vi "Sweep control.vi"(0 "Scan control":cluster{"Priority":u16, "Scan name":u16}[](array[cluster])=[{"Priority"=0, "Scan name"=1}, {"Priority"=1, "Scan name"=0}, {"Priority"=3, "Scan name"=0}, {"Priority"=2, "Scan name"=0}] {"Scan name" items=["OFF", "Vsg1", "Vsg2", "Vsgw", "Vbg", "Field", "Temp", "MW_freq", "MW_amplitude"]; "Priority" items=["Priority 0", "Priority 1", "Priority 2", "Priority 3", "Priority 4", "Priority 5"]}, 1 "Scan parameters":T2(array[cluster])=[{"DAQ Channel"=3, "Label"="\nappliedVsg=", "Scaled low"=-0.1, "Scaled high"=0.6, "Start"=-0.8, "End"=0.1, "Step"=0.001, "Scale?"=FALSE, "Output"=0}, {"DAQ Channel"=3, "Label"="\nappliedVsg2=", "Scaled low"=-0.175, "Scaled high"=0.775, "Start"=0.0, "End"=0.0, "Step"=0.01, "Scale?"=FALSE, "Output"=2}, {"DAQ Channel"=3, "Label"="\nappliedVbg=", "Scaled low"=-0.11, "Scaled high"=0.31, "Start"=-1.55, "End"=3.0, "Step"=0.015, "Scale?"=FALSE, "Output"=2}, {"DAQ Channel"=3, "Label"="\nappliedField=", "Scaled low"=-0.060000000000000005, "Scaled high"=0.14, "Start"=0.0, "End"=10000.0, "Step"=5000.0, "Scale?"=FALSE, "Output"=2}] {"Step" format="%#_6p"; "End" format="%#_6p"; "Start" format="%#_6p"; "Scaled high" format="%#_6p"; "Scaled low" format="%#_6p"}, 3 "Comments":string="SA02703G.20140721\n\nVbg=0.7V\n\nsweep Vsg2(control): -80mV to 100mV 1mV steps\n\nLockin0:18\n1: 19\n2: 21\n3: 22\n4: 23\n5: 24\n\ndrive differentially 18,24, 1mV 401mHz", 4 "Experiment folder name":string="1 - IV_sweep_Vsg") -> ()   [LabVIEW 2013]
uses:
  <userlib>/LevyLab/DAQ-Lockin-SubVI/Lockin-4461_MultiChannel - IV 3.0 globals.vi
  P:/users1/Joe/Lockin-4461_3.0 4461-4462 Multichannel Folder/DAQ-Lockin-SubVI/Lock-in Globles Multiple Inputs and Outputs.vi
panel:
  in  "OSC Configuration 2":T1(array[cluster])=[[{"Signal Type"=enum."Triangle Wave", "DC"=0.0, "Amplitude"=0.001, "frequency"=0.401, "Phase"=0.0}, {"Signal Type"=enum."Sine Wave", "DC"=0.0, "Amplitude"=0.0, "frequency"=0.401, "Phase"=0.0}], [{"Signal Type"=enum."Sine Wave", "DC"=0.0, "Amplitude"=0.0, "frequency"=0.401, "Phase"=0.0}, {"Signal Type"=enum."Sine Wave", "DC"=0.0, "Amplitude"=0.0, "frequency"=0.401, "Phase"=0.0}], [{"Signal Type"=enum."Sine Wave", "DC"=0.0, "Amplitude"=0.0, "frequency"=0.401, "Phase"=0.0}, {"Signal Type"=enum."Triangle Wave", "DC"=0.0, "Amplitude"=0.001, "frequency"=0.401, "Phase"=180.0}], [{"Signal Type"=enum."Sine Wave", "DC"=0.0, "Amplitude"=0.0, "frequency"=0.401, "Phase"=0.0}, {"Signal Type"=enum."Triangle Wave", "DC"=0.0, "Amplitude"=0.0, "frequency"=0.401, "Phase"=0.0}]] {"frequency" step=0.001 format="%.3p"; "Amplitude" format="%0.2p"; "DC" min=-0.99 max=0.99 format="%.2p"}
  in  "Additional action (indexing priority)":u16[](array[ring])=[4, 4, 4, 4] items=["Clear DAQ Tasks", "Check Temperature", "Check Field Value", "Wait", "Do Nothing"]
  in  "Number of IV curves":i32=1
  # "Instructions: \n1, you can put multiple scan names in one priority.\n2 OFF has to put in last priority"
  # "I wanted to check the temperature as well as the field (so the zero-field data isn't taken at higher temperatures) so I changed the post-action subvi slightly. In the 'check temperature' case, I made the stop condition that the temp is less than 70mK. By putting 'check temperature' with priority 1, i figure it'll set Vsg1&2 at 0, then wait for the temp to reach 70mK, before it starts sweeping prioity 0."
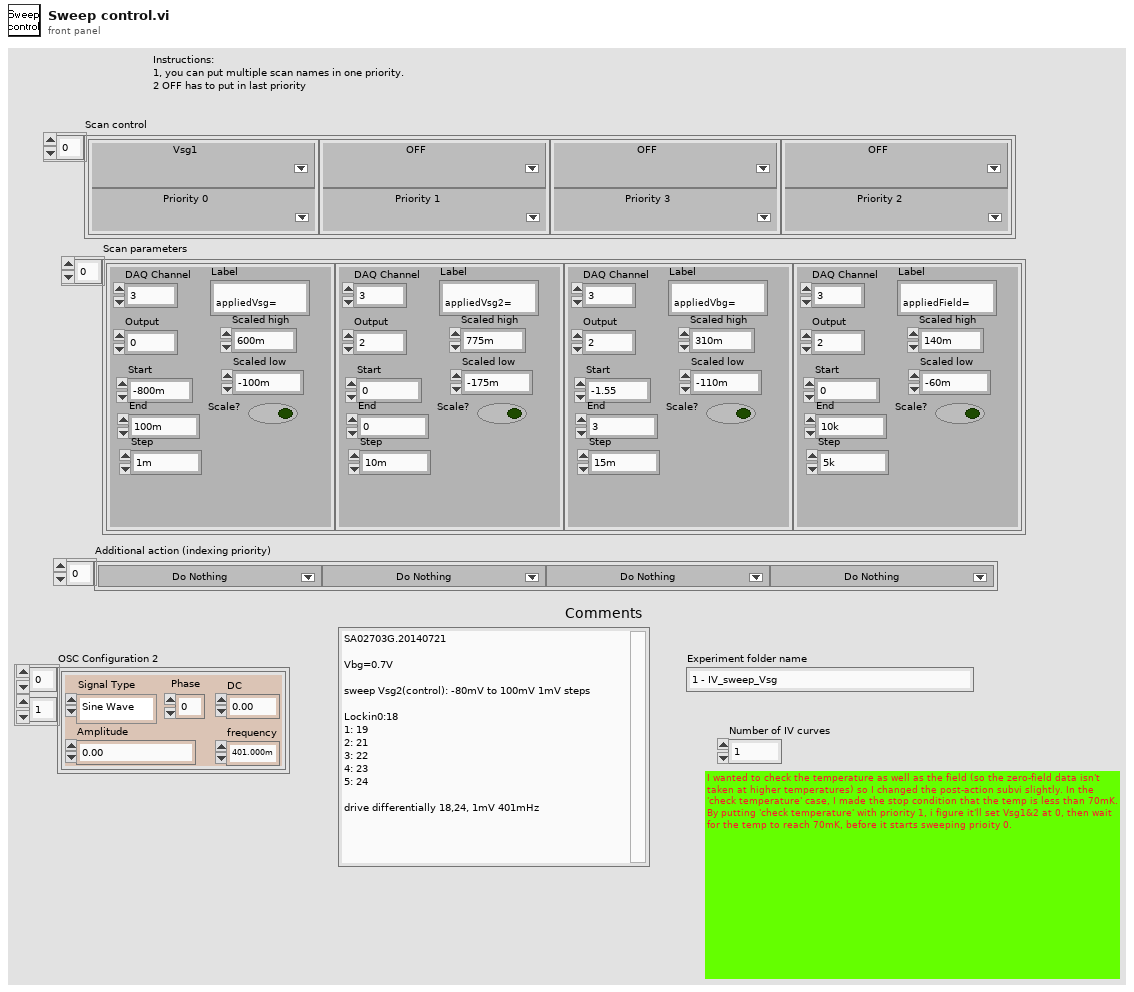
[diagram p1: front panel]
types:
  T1 = cluster{"Signal Type":enum16{"Sine Wave", "Triangle Wave", "Square Wave", "Sawtooth Wave"}, "DC":dbl, "Amplitude":dbl, "frequency":dbl, "Phase":dbl}[][]
  T2 = cluster{"DAQ Channel":i32, "Label":string, "Scaled low":dbl, "Scaled high":dbl, "Start":dbl, "End":dbl, "Step":dbl, "Scale?":bool, "Output":i32}[]
  T3 = cluster{cluster{"DAQ Channel":i32, "Label":string, "Scaled low":dbl, "Scaled high":dbl, "Start":dbl, "End":dbl, "Step":dbl, "Scale?":bool, "Output":i32}[]}[]
  T4 = cluster{cluster{"Priority":u16, "Scan name":u16}[]}[]
  T5 = cluster{cluster{"DAQ Channel":i32, "Label":string, "Scaled low":dbl, "Scaled high":dbl, "Start":dbl, "End":dbl, "Step":dbl, "Scale?":bool, "Output":i32}[]}
  T6 = cluster{cluster{"Priority":u16, "Scan name":u16}[]}
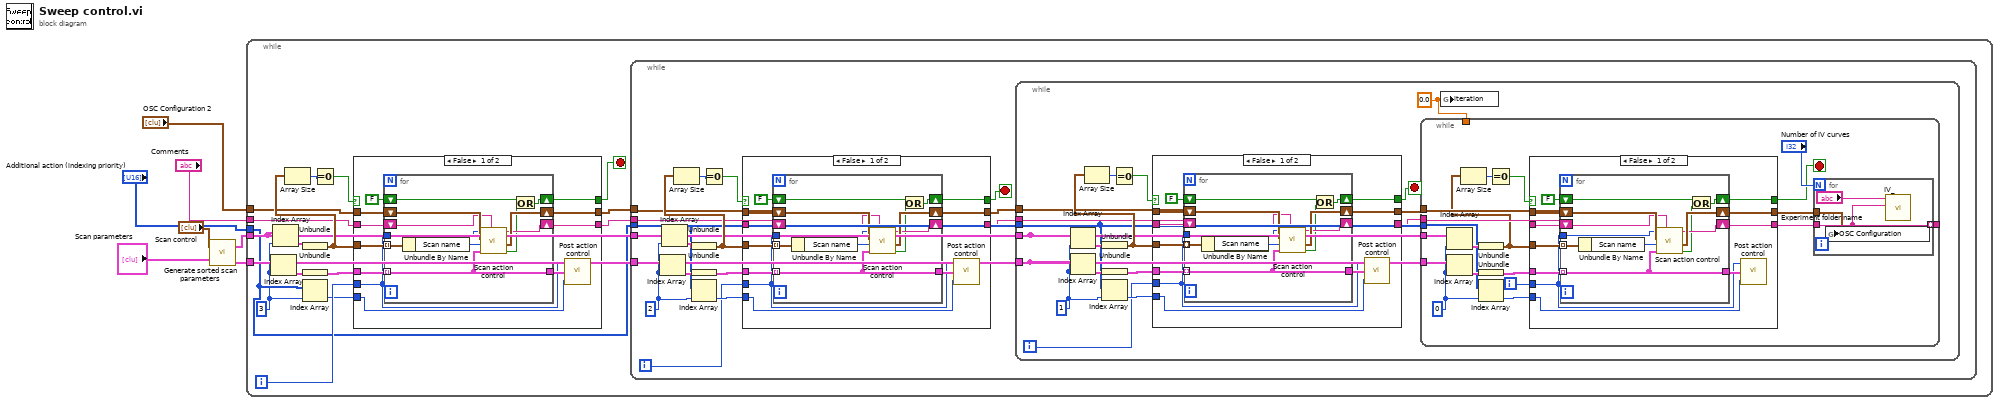
[diagram p0: block diagram]
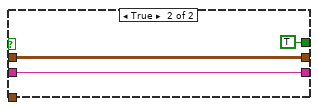
[diagram p2: hidden frame]
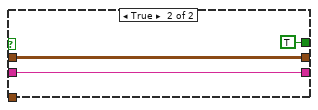
[diagram p3: hidden frame]
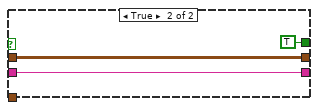
[diagram p4: hidden frame]
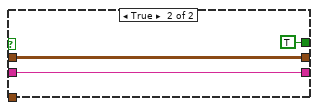
[diagram p5: hidden frame]
diagram:
  n1 = call <userlib>:"Generate sorted scan parameters.vi"("Scan parameters 2"="Scan parameters", "Scan control"="Scan control") -> ("Sorted scan parameters"=w4:T3, "Sorted scan control"=w3:T4)
  n2 = while {
    tunnel: "Comments" -> [w11]
    tunnel: "OSC Configuration 2" -> [w12]
    tunnel: w4 -> [w19]
    tunnel: w3 -> [w18]
    tunnel: "Additional action (indexing priority)" -> [w13]
    i -> [w15]
    stop <- w16 stop-if-true
    w8 = 3
    n3 = Index Array(array=w19, index=w8) -> (element=w20:T5)
    n4 = Index Array(array=w18, index=w8) -> (element=w17:T6)
    n5 = Unbundle(w17) -> (w22:cluster{"Priority":u16, "Scan name":u16}[])
    n6 = Array Size(array=w22) -> (size(s)=w23:i32)
    n7 = Unbundle(w20) -> (w21:T2)
    n8 = Index Array(array=w13, index=w8) -> (element=w14:u16)
    n9 = Equal To 0?(x=w23) -> (x = 0?=w24:bool)
    n10 = case shown="False" w24 {
      tunnel: w21 -> [w35 _]
      tunnel: [w34 w48] -> w10
      tunnel: [w33 w47] -> w9
      tunnel: [w27 TRUE ("Stop?")] -> w16
      tunnel: w22 -> [w32 _]
      tunnel: w15 -> [w29 _]
      tunnel: w14 -> [w30 _]
      tunnel: w12 -> [w26 w48]
      tunnel: w11 -> [w25 w47]
      frame False {
        n11 = for {
          tunnel: w32 -> [w46] mode=indexing
          tunnel: w35 -> [w39] mode=indexing
          tunnel: w29 -> [w40]
          shift-right: [w44] -> w34
          shift-left: w26 -> [w43]
          shift-right: [w42] -> w33
          shift-left: w25 -> [w41]
          tunnel: [w39] -> w31
          shift-right: [w36] -> w27
          shift-left: FALSE -> [w38]
          n12 = Unbundle By Name(w46) -> ("Scan name"=w45:u16)
          n13 = call <userlib>:"Scan action control.vi"("Comments"=w41, "Scan Parameters"=w39, "Scan control"=w45, "OSC Configuration 2"=w43, "Index"=w40) -> ("Stop?"=w37:bool, "OSC Configuration 3"=w44:T1, "Comments out"=w42:string)  [unwired: 2 in]
          n14 = Or(x=w38, y=w37) -> (x .or. y?=w36:bool)
        }
        n15 = call <userlib>:"Post action control.vi"("Action"=w30, "Scan Parameters"=w31, "Index"=w29) -> ()  [unwired: 1 out]
      }
      frame True {
      }
    }
    n16 = while {
      tunnel: w19 -> [w59]
      tunnel: w18 -> [w58]
      tunnel: w13 -> [w57]
      tunnel: w9 -> [w56]
      tunnel: w10 -> [w55]
      i -> [w54]
      stop <- w53 stop-if-true
      w50 = 2
      n17 = Index Array(array=w59, index=w50) -> (element=w65:T5)
      n18 = Index Array(array=w58, index=w50) -> (element=w66:T6)
      n19 = Unbundle(w66) -> (w63:cluster{"Priority":u16, "Scan name":u16}[])
      n20 = Array Size(array=w63) -> (size(s)=w61:i32)
      n21 = Unbundle(w65) -> (w64:T2)
      n22 = Index Array(array=w57, index=w50) -> (element=w62:u16)
      n23 = Equal To 0?(x=w61) -> (x = 0?=w60:bool)
      n24 = case shown="False" w60 {
        tunnel: w64 -> [w77 _]
        tunnel: w55 -> [w76 w91]
        tunnel: w56 -> [w75 w90]
        tunnel: [w74 w91] -> w52
        tunnel: [w73 w90] -> w51
        tunnel: [w67 TRUE ("Stop?")] -> w53
        tunnel: w63 -> [w72 _]
        tunnel: w54 -> [w69 _]
        tunnel: w62 -> [w70 _]
        frame False {
          n25 = for {
            tunnel: w72 -> [w88] mode=indexing
            tunnel: w77 -> [w81] mode=indexing
            tunnel: w69 -> [w82]
            shift-right: [w86] -> w74
            shift-left: w76 -> [w85]
            shift-right: [w84] -> w73
            shift-left: w75 -> [w83]
            tunnel: [w81] -> w71
            shift-right: [w78] -> w67
            shift-left: FALSE -> [w80]
            n26 = Unbundle By Name(w88) -> ("Scan name"=w87:u16)
            n27 = call <userlib>:"Scan action control.vi"("Comments"=w83, "Scan Parameters"=w81, "Scan control"=w87, "OSC Configuration 2"=w85, "Index"=w82) -> ("Stop?"=w79:bool, "OSC Configuration 3"=w86:T1, "Comments out"=w84:string)  [unwired: 2 in]
            n28 = Or(x=w80, y=w79) -> (x .or. y?=w78:bool)
          }
          n29 = call <userlib>:"Post action control.vi"("Action"=w70, "Scan Parameters"=w71, "Index"=w69) -> ()  [unwired: 1 out]
        }
        frame True {
        }
      }
      n30 = while {
        tunnel: w52 -> [w101]
        tunnel: w51 -> [w100]
        tunnel: w58 -> [w99]
        tunnel: w59 -> [w98]
        tunnel: w57 -> [w97]
        i -> [w96]
        stop <- w93 stop-if-true
        w92 = 1
        w109 = 0.0 ("iteration")
        n31 = Index Array(array=w99, index=w92) -> (element=w102:T6)
        n32 = Index Array(array=w98, index=w92) -> (element=w103:T5)
        n33 = Unbundle(w102) -> (w105:cluster{"Priority":u16, "Scan name":u16}[])
        n34 = Array Size(array=w105) -> (size(s)=w107:i32)
        n35 = Unbundle(w103) -> (w104:T2)
        n36 = Index Array(array=w97, index=w92) -> (element=w106:u16)
        n37 = Equal To 0?(x=w107) -> (x = 0?=w108:bool)
        n38 = case shown="False" w108 {
          tunnel: w104 -> [w120 _]
          tunnel: w101 -> [w119 w134]
          tunnel: w100 -> [w118 w133]
          tunnel: [w117 w134] -> w94
          tunnel: [w116 w133] -> w95
          tunnel: [w110 TRUE ("Stop?")] -> w93
          tunnel: w105 -> [w115 _]
          tunnel: w96 -> [w112 _]
          tunnel: w106 -> [w113 _]
          frame False {
            n39 = for {
              tunnel: w115 -> [w131] mode=indexing
              tunnel: w120 -> [w124] mode=indexing
              tunnel: w112 -> [w125]
              shift-right: [w129] -> w117
              shift-left: w119 -> [w128]
              shift-right: [w127] -> w116
              shift-left: w118 -> [w126]
              tunnel: [w124] -> w114
              shift-right: [w121] -> w110
              shift-left: FALSE -> [w123]
              n40 = Unbundle By Name(w131) -> ("Scan name"=w130:u16)
              n41 = call <userlib>:"Scan action control.vi"("Comments"=w126, "Scan Parameters"=w124, "Scan control"=w130, "OSC Configuration 2"=w128, "Index"=w125) -> ("Stop?"=w122:bool, "OSC Configuration 3"=w129:T1, "Comments out"=w127:string)  [unwired: 2 in]
              n42 = Or(x=w123, y=w122) -> (x .or. y?=w121:bool)
            }
            n43 = call <userlib>:"Post action control.vi"("Action"=w113, "Scan Parameters"=w114, "Index"=w112) -> ()  [unwired: 1 out]
          }
          frame True {
          }
        }
        n44 = while {
          tunnel: w99 -> [w152]
          tunnel: w98 -> [w151]
          tunnel: w94 -> [w147]
          tunnel: w95 -> [w146]
          tunnel: w97 -> [w140]
          tunnel: w109 -> [_]
          tunnel: [w136] -> _
          i -> [w141]
          stop <- w143 stop-if-true
          w135 = 0
          n45 = Index Array(array=w152, index=w135) -> (element=w150:T6)
          n46 = Index Array(array=w151, index=w135) -> (element=w149:T5)
          n47 = Unbundle(w150) -> (w142:cluster{"Priority":u16, "Scan name":u16}[])
          n48 = Array Size(array=w142) -> (size(s)=w138:i32)
          n49 = Unbundle(w149) -> (w148:T2)
          n50 = Index Array(array=w140, index=w135) -> (element=w139:u16)
          n51 = Equal To 0?(x=w138) -> (x = 0?=w137:bool)
          n52 = case shown="False" w137 {
            tunnel: w148 -> [w164 _]
            tunnel: w147 -> [w163 w178]
            tunnel: w146 -> [w162 w177]
            tunnel: [w161 w178] -> w145
            tunnel: [w160 w177] -> w144
            tunnel: [w154 TRUE ("Stop?")] -> w143
            tunnel: w142 -> [w159 _]
            tunnel: w141 -> [w156 _]
            tunnel: w139 -> [w157 _]
            frame False {
              n53 = for {
                tunnel: w159 -> [w175] mode=indexing
                tunnel: w164 -> [w168] mode=indexing
                tunnel: w156 -> [w169]
                shift-right: [w173] -> w161
                shift-left: w163 -> [w172]
                shift-right: [w171] -> w160
                shift-left: w162 -> [w170]
                tunnel: [w168] -> w158
                shift-right: [w165] -> w154
                shift-left: FALSE -> [w167]
                n54 = Unbundle By Name(w175) -> ("Scan name"=w174:u16)
                n55 = call <userlib>:"Scan action control.vi"("Comments"=w170, "Scan Parameters"=w168, "Scan control"=w174, "OSC Configuration 2"=w172, "Index"=w169) -> ("Stop?"=w166:bool, "OSC Configuration 3"=w173:T1, "Comments out"=w171:string)  [unwired: 2 in]
                n56 = Or(x=w167, y=w166) -> (x .or. y?=w165:bool)
              }
              n57 = call <userlib>:"Post action control.vi"("Action"=w157, "Scan Parameters"=w158, "Index"=w156) -> ()  [unwired: 1 out]
            }
            frame True {
            }
          }
          n58 = for {
            N: "Number of IV curves" -> [_]
            tunnel: w145 -> [w179]
            tunnel: w144 -> [w180]
            tunnel: [w180] -> w136 mode=indexing
            n59 = global write "Lock-in Globles Multiple Inputs and Outputs.vi" "OSC Configuration"(w179) -> ()
            n60 = call "IV_.vi"("Notes"=w180, "Experiment folder name"="Experiment folder name") -> ()  [unwired: 10 in]
          }
        }
        n61 = global write "Lockin-4461_MultiChannel - IV 3.0 globals.vi" "iteration"(w109) -> ()
      }
    }
  }
